vi "AutoRunEngine.vi"(6 "Stop":bool, 7 "Comms in cluster":T3={"Lakeshore port"="COM6", "Lakeshore Error"={"status"=FALSE, "code"=0, "source"=""}, "Cernox Channel"=17, "Sample Channel "=1, "Arduino port \n(for magnetic poles)"="COM3", "Switchboard port"="USB0::0x05E6::0x3706::04089883::INSTR", "Switchboard Error"={"status"=FALSE, "code"=0, "source"=""}, "Hall probe/Aux"=FALSE} {"Cernox Channel" items=["1"=1, "2"=2, "3"=3, "4"=4, "5"=5, "6"=6, "7"=7, "8"=8, "9"=9, "10"=10, "11"=11, "12"=12, "13"=13, "14"=14, "15"=15, "16"=16, "A"=17]; "Sample Channel" items=["1"=1, "2"=2, "3"=3, "4"=4, "5"=5, "6"=6, "7"=7, "8"=8, "9"=9, "10"=10, "11"=11, "12"=12, "13"=13, "14"=14, "15"=15, "16"=16, "A (Control Input)"=17]}, 8 "Save Data":bool, 9 "File path":path) -> (1 "Comms out cluster":T1={"Lakeshore port"="COM6", "Lakeshore Error"={"status"=FALSE, "code"=0, "source"=""}, "Cernox Channel"="", "Sample Channel "="", "Arduino port \n(for magnetic poles)"="COM3", "Switchboard port"="USB0::0x05E6::0x3706::04089883::INSTR", "Switchboard Error 2"={"status"=FALSE, "code"=0, "source"=""}}, 2 "Graph indices out":dbl[](array[numeric]), 3 "Array":dbl[][](array[numeric]))   [LabVIEW 2017, in "Fridge Software v2.1.lvlib"]
uses:
  Fridge Software v2.1.lvlib
  <vilib>/Platform/TimedLoop/XDataNode/timing_clust.ctl
  <vilib>/Platform/TimedLoop/XDataNode/nitl_modes.ctl
  <vilib>/Platform/TimedLoop/XDataNode/wakeup.ctl
  <vilib>/Utility/file.llb/Write Delimited Spreadsheet (DBL).vi
  <vilib>/platform/TimedLoop/XDataNode/XDataNode.xnode
  <instrlib>/Lake Shore 372/Lake Shore 372.lvlib
  <instrlib>/Keithley 3706/Keithley 3700 Series.lvlib
  <vilib>/Platform/TimedLoop/XDataNode/XDNodeRunTimeDep.lvlib
panel:
  out "Input Reading Status Query":string
  out "Elapsed time":dbl=500.0 min=50.0 step=100.0
  out "Magnetic Poles \nLive  Voltage":dbl format="%#_5g"
  in  "Measurement\nperiod":i64=500 min=100 step=100
  out "Power Reading":dbl min=0.0 max=0.01 step=1e-05 format="%^.3g"
  out "Sample Reactance":dbl min=0.0 max=63200000.0 step=1e-05 format="%.3g"
  out "Cernox Resistance":dbl min=0.0 max=63200000.0 step=1e-05 format="%.3g"
  in  "R(T,H) tab":enum32{"R(T)", "R(H)"}(tab)
  in  "Clear R(T) graph":bool
  in  "Autoscale R(T)":bool=TRUE caption="Autoscale"
  out "R(T) Graph":cluster{dbl[], dbl[]}(graph)
  in  "Clear H(T) graph":bool
  in  "Autoscale H(T)":bool=TRUE caption="Autoscale"
  out "R(H) Graph":cluster{dbl[], dbl[]}(graph)
  in  "Clear H(t) graph":bool
  in  "Clear T(t) graph":bool
  in  "Clear R(t) graph":bool
  out "Sample Resistance":dbl min=0.0 max=63200000.0 step=1e-05 format="%^.5g"
  out "Cernox Temperature":dbl min=0.0 max=1000.0 step=1e-05 format="%.4f"
  in  "Autoscale H(t)":bool=TRUE caption="Autoscale"
  in  "Autoscale T(t)":bool=TRUE caption="Autoscale"
  in  "Autoscale R(t)":bool=TRUE caption="Autoscale"
  out "H(t) Graph 4":cluster{dbl[], dbl[]}(graph)
  out "T(t) Graph 3":cluster{dbl[], dbl[]}(graph)
  out "R(t) Graph":cluster{dbl[], dbl[]}(graph)
  in  "Measurement":T2(tab)
  in  "Update":bool
  out "Excitation  Ind":bool=TRUE
  out "Excitation Mode Ind":u16(ring)=1 items=["Voltage", "Current"]
  out "Excitation Range Ind":u16(ring)=19 items=["31.6 mA"=22, "10.0 mA"=21, "3.16 mA"=20, "1.00 mA"=19, "316 uA"=18, "100 uA"=17, "31.6 uA"=16, "10.0 uA"=15, "3.16 uA"=14, "1.00 uA"=13, "632 mV / 316 nA"=12, "200 mV / 100 nA"=11, "63.2 mV / 31.6 nA"=10, "20.0 mV / 10.0 nA"=9, "6.32 mV / 3.16 nA"=8, "2.00 mV / 1.00 nA"=7, "632 uV / 316 pA"=6, "200 uV / 100 pA"=5, "63.2 uV / 31.6 pA"=4, "20.0 uV / 10.0 pA"=3, "6.32 uV / 3.16 pA"=2, "2.00 uV / 1.00 pA"=1]
  out "Autorange Ind":u16(ring) items=["Autorange off", "Autorange Current", "ROX 102B Autorange"]
  out "Resistance Range Ind":u16(ring)=8 items=["63.2 MOhm"=22, "20.0 MOhm"=21, "6.32 MOhm"=20, "2.00 MOhm"=19, "632 kOhm"=18, "200 kOhm"=17, "63.2 kOhm"=16, "20.0 kOhm"=15, "6.32 kOhm"=14, "2.00 kOhm"=13, "632 Ohm"=12, "200 Ohm"=11, "63.2 Ohm"=10, "20.0 Ohm"=9, "6.32 Ohm"=8, "2.00 Ohm"=7, "632 mOhm"=6, "200 mOhm"=5, "63.2 mOhm"=4, "20.0 mOhm"=3, "6.32 mOhm"=2, "2.00 mOhm"=1]
  out "Preferred Units Ind":u16(ring)=2 items=["Kelvin"=1, "Ohms"=2]
  out "Temperature Limit Ind":dbl min=0.0 max=2999.0 step=1.0
  in  "Excitation Mode":u16(ring)=1 items=["Voltage", "Current"]
  in  "Excitation Range":u16(ring)=19 items=["31.6 mA"=22, "10.0 mA"=21, "3.16 mA"=20, "1.00 mA"=19, "316 uA"=18, "100 uA"=17, "31.6 uA"=16, "10.0 uA"=15, "3.16 uA"=14, "1.00 uA"=13, "632 mV / 316 nA"=12, "200 mV / 100 nA"=11, "63.2 mV / 31.6 nA"=10, "20.0 mV / 10.0 nA"=9, "6.32 mV / 3.16 nA"=8, "2.00 mV / 1.00 nA"=7, "632 uV / 316 pA"=6, "200 uV / 100 pA"=5, "63.2 uV / 31.6 pA"=4, "20.0 uV / 10.0 pA"=3, "6.32 uV / 3.16 pA"=2, "2.00 uV / 1.00 pA"=1]
  in  "Autorange (0: Autorange off)":u16(ring) items=["Autorange off", "Autorange Current", "ROX 102B Autorange"]
  in  "Resistance Range":u16(ring)=8 items=["63.2 MOhm"=22, "20.0 MOhm"=21, "6.32 MOhm"=20, "2.00 MOhm"=19, "632 kOhm"=18, "200 kOhm"=17, "63.2 kOhm"=16, "20.0 kOhm"=15, "6.32 kOhm"=14, "2.00 kOhm"=13, "632 Ohm"=12, "200 Ohm"=11, "63.2 Ohm"=10, "20.0 Ohm"=9, "6.32 Ohm"=8, "2.00 Ohm"=7, "632 mOhm"=6, "200 mOhm"=5, "63.2 mOhm"=4, "20.0 mOhm"=3, "6.32 mOhm"=2, "2.00 mOhm"=1]
  in  "Preferred Units (2: Ohms)":u16(ring)=2 items=["Kelvin"=1, "Ohms"=2]
  in  "Temperature Limit (0 Kelvin)":dbl min=0.0 max=2999.0 step=1.0
  in  "Excitation  (T: On)":bool=TRUE caption="On\n\nOff"
  in  "Grab settings":bool
  in  "Heater Setpoint":dbl
  out "Heater Setpoint Ind":string
  in  "Grab Heater settings":bool
  in  "Update Heater Settings":bool
  in  "I+":i32 min=0 max=24 step=1
  in  "I-":i32 min=0 max=24 step=1
  in  "V+":i32 min=0 max=24 step=1
  in  "V-":i32 min=0 max=24 step=1
  in  "Close pins (safe)":bool caption="Close I-V pins -> Lift ground -> Lift common -> Current on"
  in  "Lift pins (safe)":bool caption="Current off -> Common closed -> Ground -> Lift I-V pins"
  in  "Channel Open/Close Array":string
  in  "Open":bool
  in  "Close":bool
  in  "Open All IV":bool
  out "Closed Channels":string
  out "Ground closed":bool
  out "Common rail \nclosed":bool
  out "Common-ground \nlink closed":bool
  in  "Append file":bool
  in  "Aux max voltage (mV)":dbl
  in  "Aux Field Range (Oe)":dbl
  # "Created by Daniel Bromley & Alex Wright, IPF Ltd 2021"
  # "Lakeshore - Measurement"
  # "Channels:"
  # "Keithley - Switchboard"
  # "s"
  # "V"
  # "ms"
  # "W"
  # "jW"
  # "W"
  # "W"
  # "K"
  # "Lakeshore - Measurement"
  # "Channels:"
  # "Keithley - Switchboard"
  # "Hall probe"
  # "Aux"
  # "Excitation Mode"
  # "Excitation Range"
  # "Autorange"
  # "Resistance Range"
  # "Preferred Units"
  # "Temperature Limit"
  # "Excitation"
  # "IV pins"
  # "Array"
  # "Set Filename and Path"
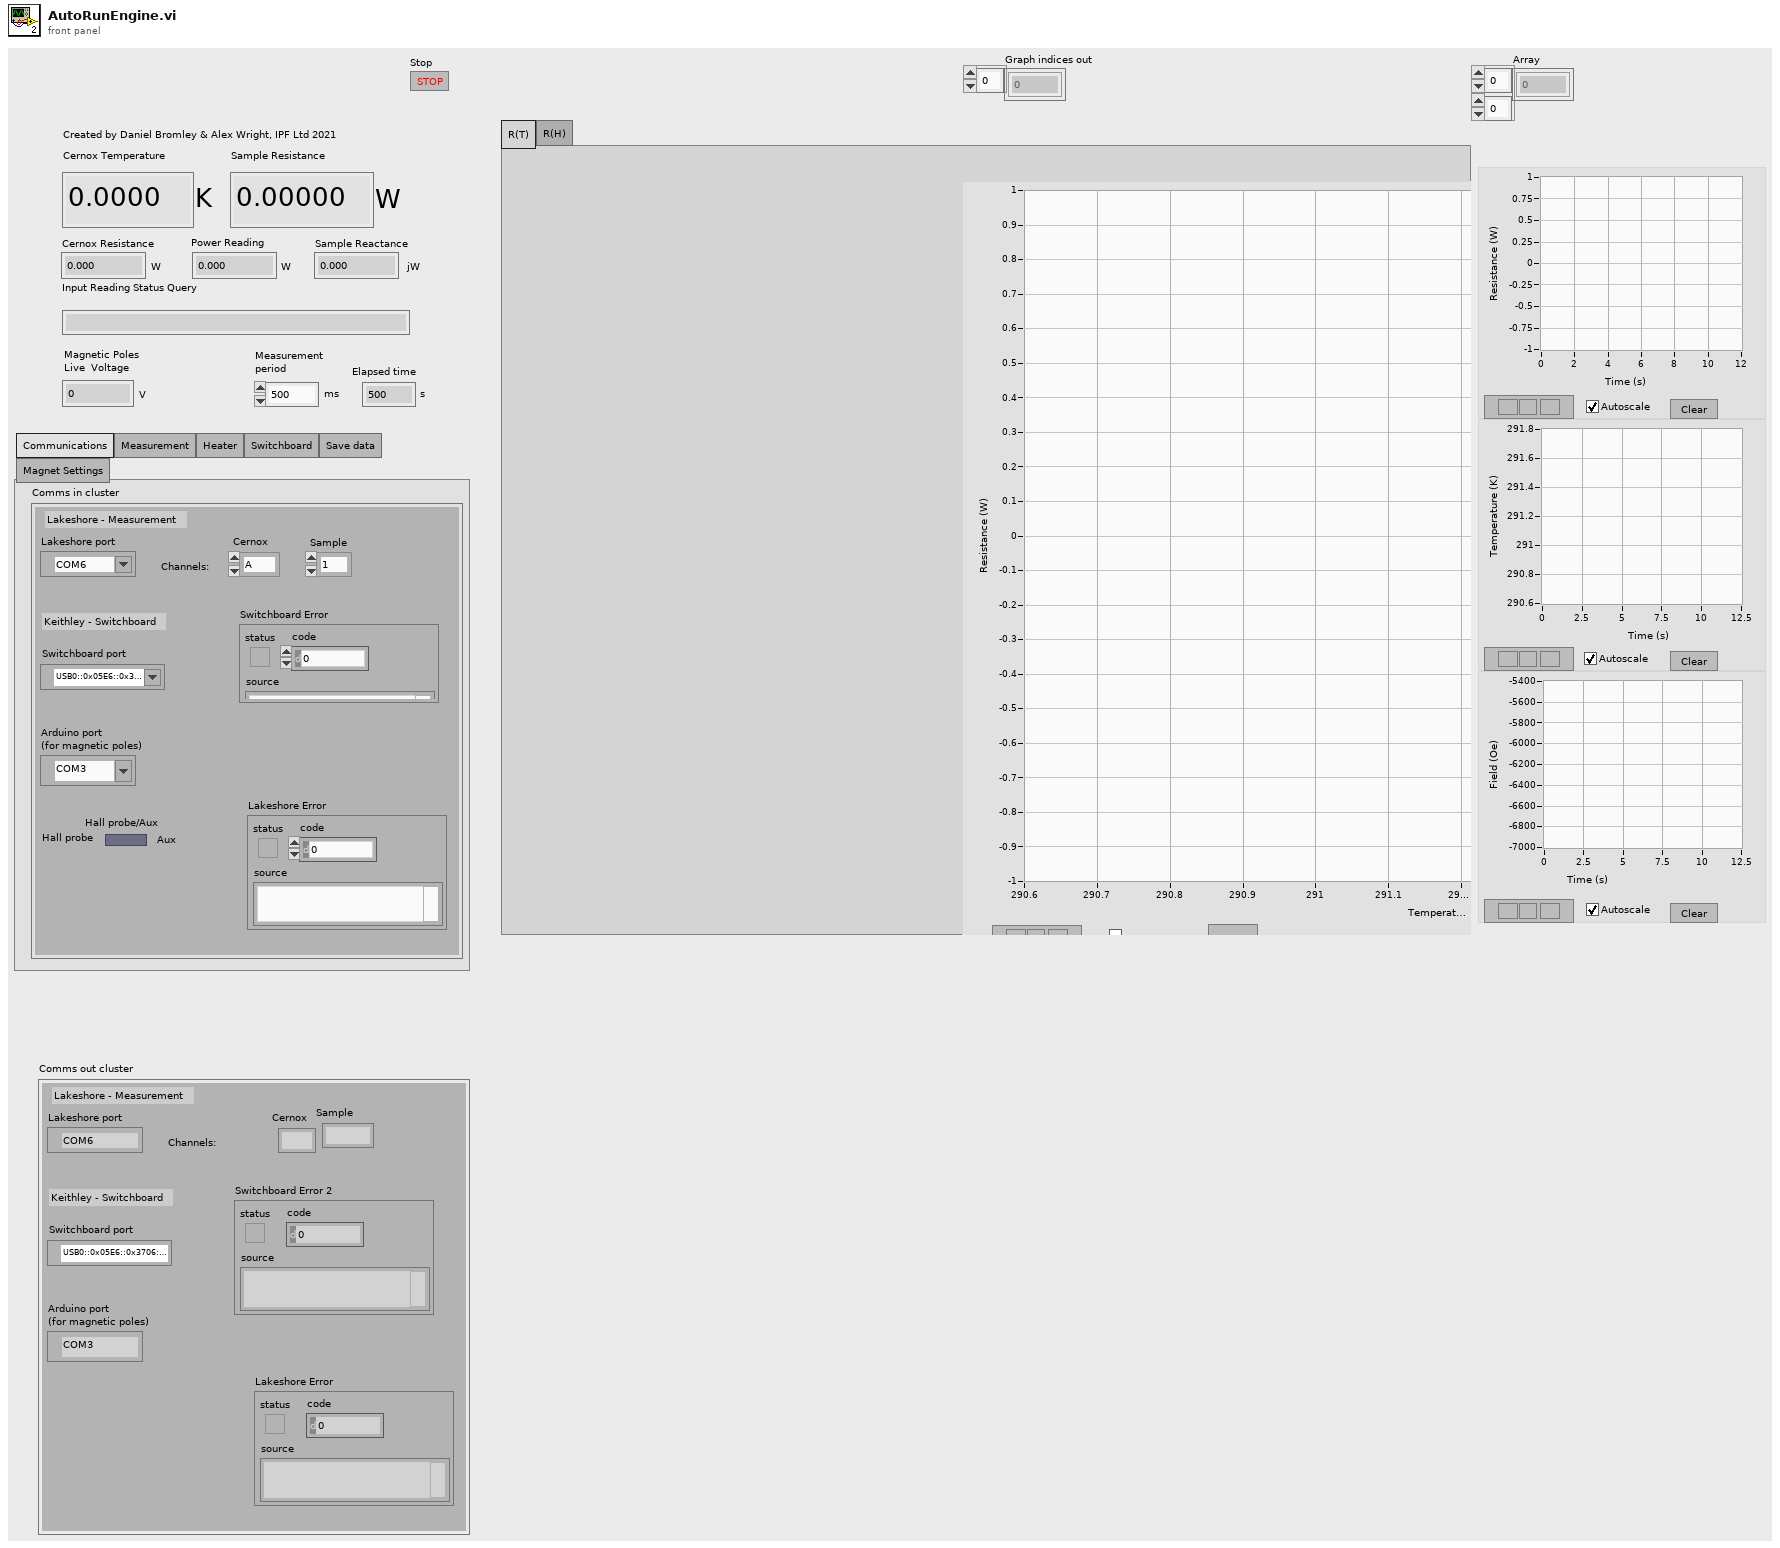
[diagram p1: front panel]
types:
  T1 = cluster{"Lakeshore port":refnum<visa-resource-name>, "Lakeshore Error":errorcluster, "Cernox Channel":string, "Sample Channel ":string, "Arduino port \n(for magnetic poles)":refnum<visa-resource-name>, "Switchboard port":refnum<visa-resource-name>, "Switchboard Error 2":errorcluster}
  T2 = enum32{"Communications", "Measurement", "Heater", "Switchboard", "Save data", "Magnet Settings"}
  T3 = cluster{"Lakeshore port":refnum<visa-resource-name>, "Lakeshore Error":errorcluster, "Cernox Channel":u16, "Sample Channel ":u16, "Arduino port \n(for magnetic poles)":refnum<visa-resource-name>, "Switchboard port":refnum<visa-resource-name>, "Switchboard Error":errorcluster, "Hall probe/Aux":bool}
  T4 = typedef "XDNodeRunTimeDep.lvlib/timing_clust.ctl" = cluster{"Expected End [f-1]":u64, "Actual End [f-1]":u64, "Finished Late? [f-1]":bool, "Expected End [i-1]":u64, "Actual End [i-1]":u64, "Finished Late? [i-1]":bool, "Expected Start [i]":u64, "Actual Start [i]":u64, "Expected Start [f]":u64, "Actual Start [f]":u64, "Source Name":string, "Structure Name":string, "Period":i64, "Deadline":i64, "Offset":i64, "Start":i64, "Priority":i32, "Timeout":i32, "Mode":T5, "Wakeup Reason":T6, "Error":errorcluster, "Source Type":string, "Secondary Source Type":string, "Global End Time":u64, "Global Start Time":u64, "Frame Duration":u64, "Iteration Duration":u64, "Assigned CPU":i32, "I/O Scan Engine Mode":u32}
  T5 = typedef "XDNodeRunTimeDep.lvlib/nitl_modes.ctl" = enum32{"No Change", "Process missed periods, maintain original phase", "Discard missed periods, maintain original phase", "Process missed periods, ignore original phase", "Discard missed periods, ignore original phase"}
  T6 = typedef "XDNodeRunTimeDep.lvlib/wakeup.ctl" = enum32{"Normal", "Aborted", "Asynchronous wakeup", "Timing source error", "Timed loop error", "Timeout"}
  T7 = typedef "eventsource.ctl" = u32
  T8 = typedef "lveventtype.ctl" = enum32{"Null", "Timeout", "Annotation Menu Selection", "Annotation Menu Selection?", "App Instance Close", "App Instance Close?", "Autoscale Range Change", "Bookmark Info Change", "Cell Edit", "Cell Edit?", "Cursor Grab", "Cursor Grab?", "Cursor Menu Selection", "Cursor Menu Selection?", "Cursor Move", "Cursor Release", "Data Change", "Direction Change", "Display State Change", "Drag Ended", "Drag Enter", "Drag Leave", "Drag Over", "Drag Source Update", "Drag Starting", "Drag Starting?", "Drop", "Exec State Change", "Key Down", "Key Down?", "Key Repeat", "Key Repeat?", "Key Up", "Listbox Double Click", "Menu Activation?", "Menu Selection (App)", "Menu Selection? (App)", "Menu Selection (User)", "Mouse Down", "Mouse Down?", "Mouse Enter", "Mouse Leave", "Mouse Move", "Mouse Up", "Mouse Wheel", "NI Security User Change (App)", "Pane Size", "Panel Close", "Panel Close?", "Panel Resize", "Plot Attribute Change", "Scale Range Change", "Shortcut Menu Activation?", "Shortcut Menu Selection (App)", "Shortcut Menu Selection? (App)", "Shortcut Menu Selection (User)", "Tree Double Click", "Tree Drag", "Tree Drag?", "Tree Drop", "Tree Drop?", "Tree Item Close", "Tree Item Close?", "Tree Item Open", "Tree Item Open?", "User Event", "Value Change"}
  T9 = cluster{"VISA Refnum out":refnum<visa-resource-name>, "error out":errorcluster, "Channel Str":string, "Channel Str":string, "VISA Refnum out":refnum<visa-resource-name>, "VISA resource name out":refnum<visa-resource-name>, "error out":errorcluster}
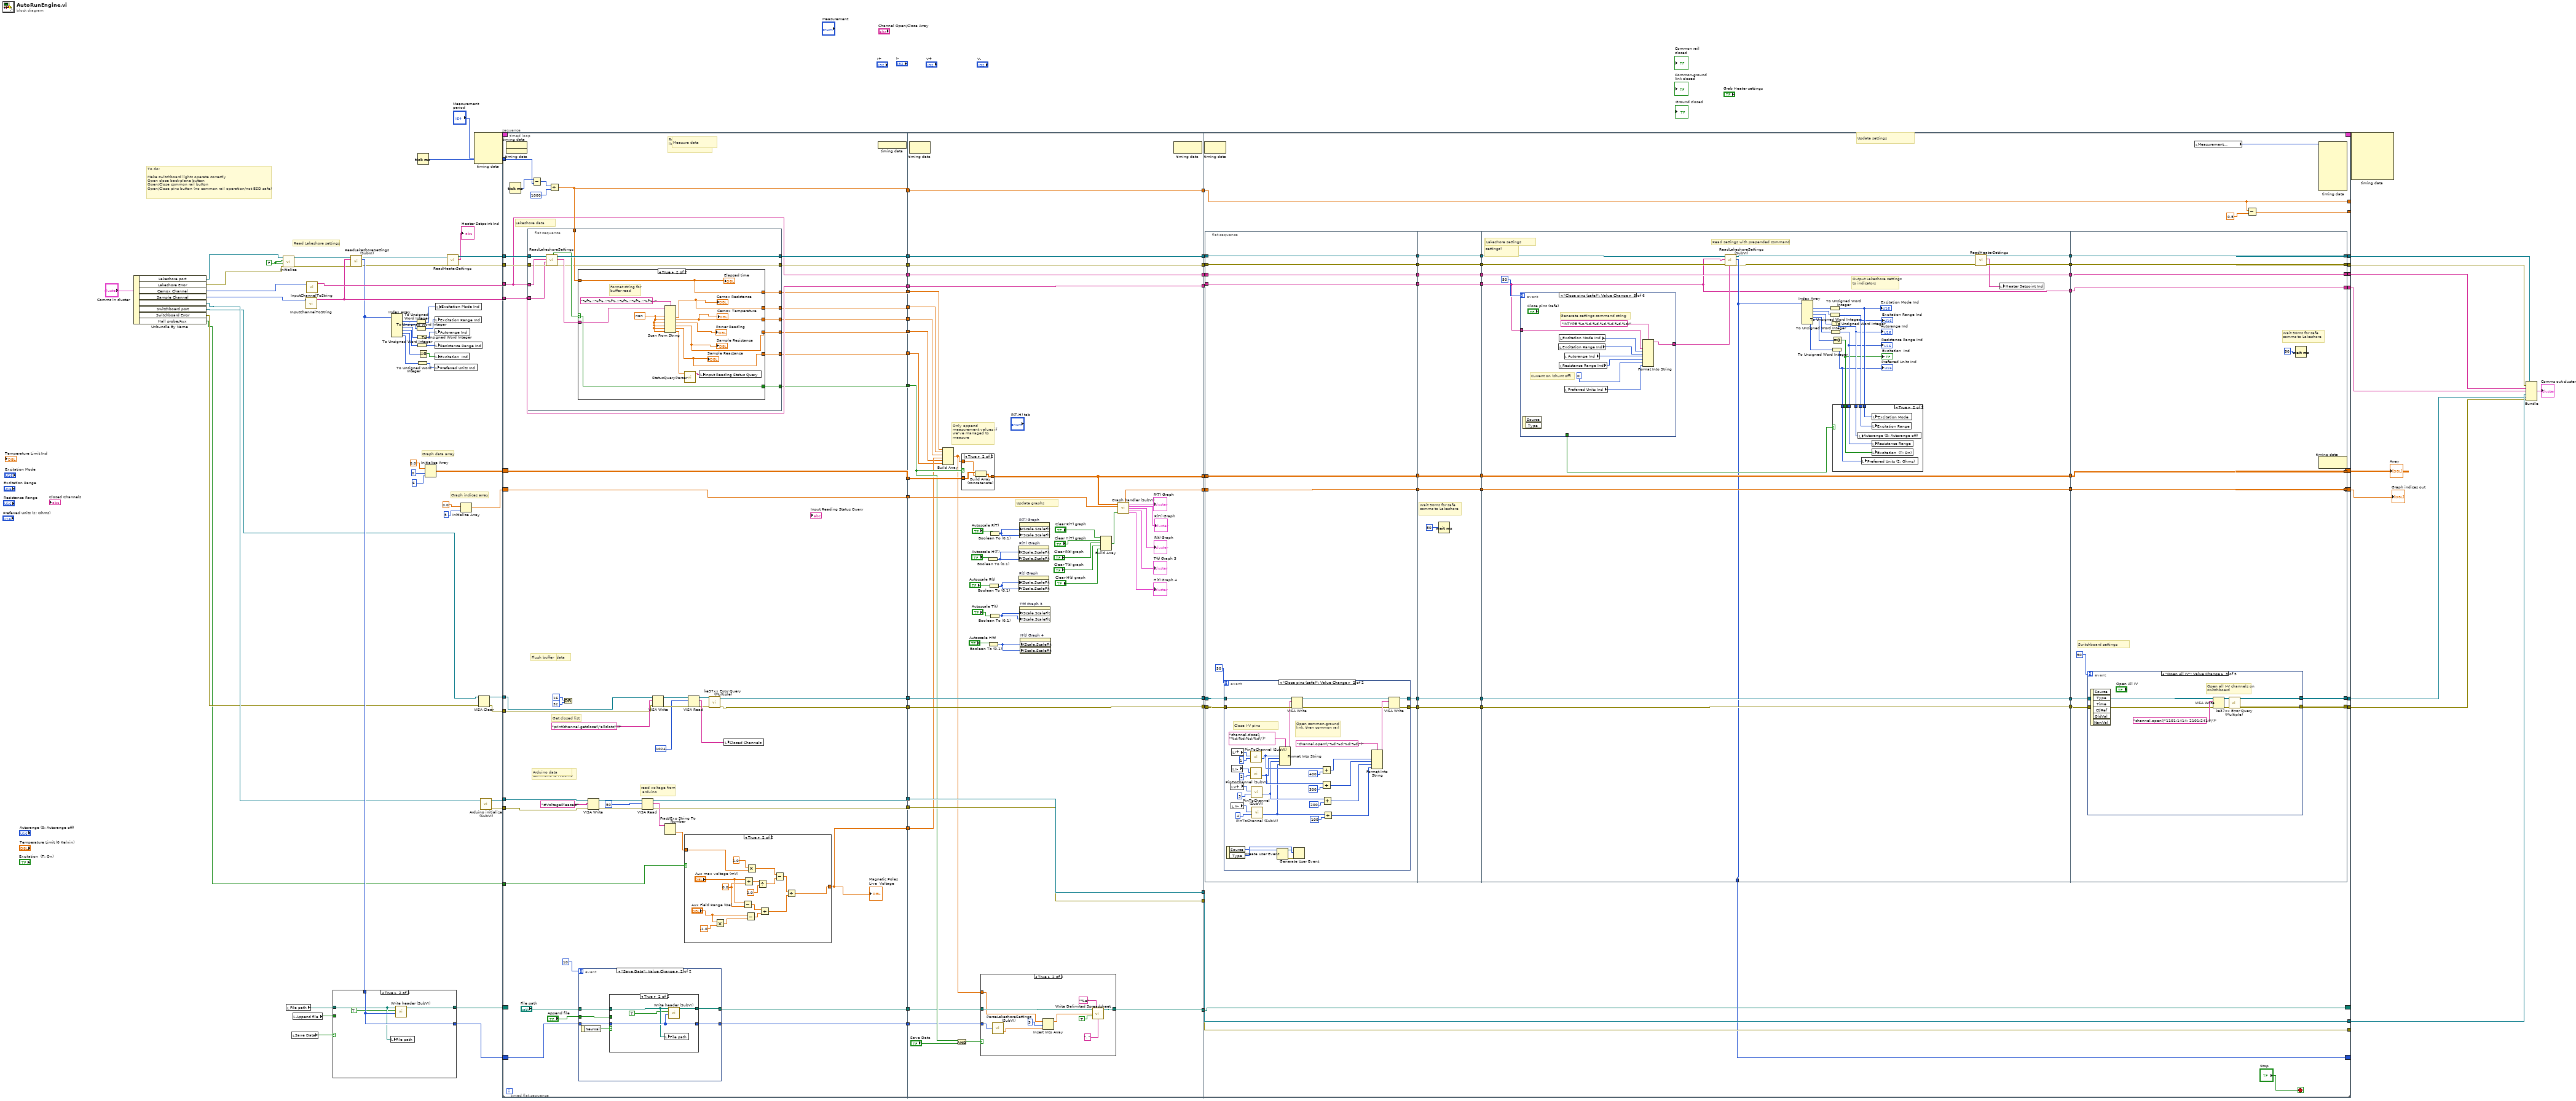
[diagram p0: block diagram]
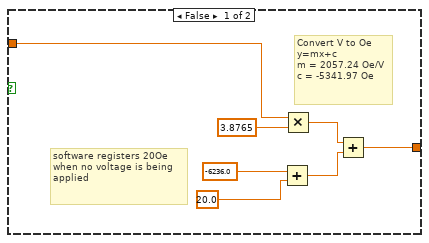
[diagram p3: hidden frame]
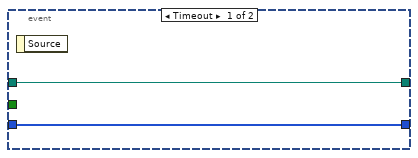
[diagram p4: hidden frame]
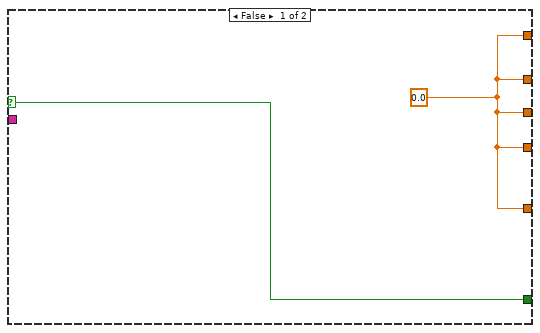
[diagram p6: hidden frame]
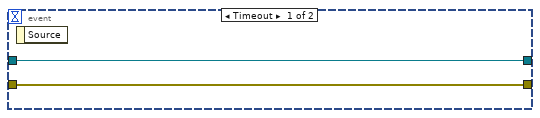
[diagram p9: hidden frame]
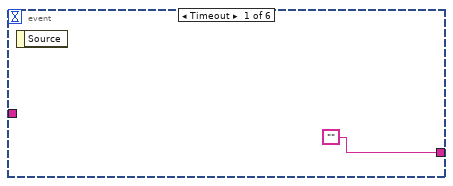
[diagram p10: hidden frame]
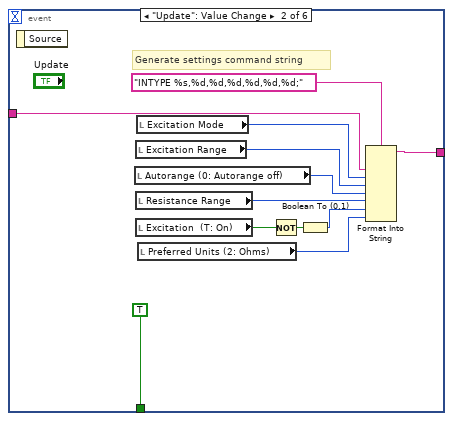
[diagram p11: hidden frame]
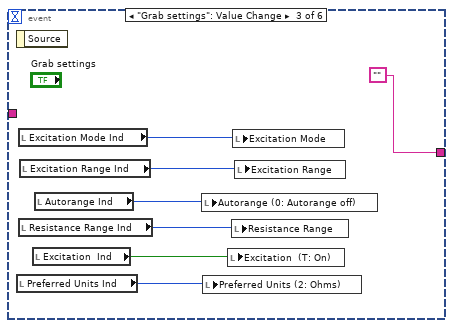
[diagram p12: hidden frame]
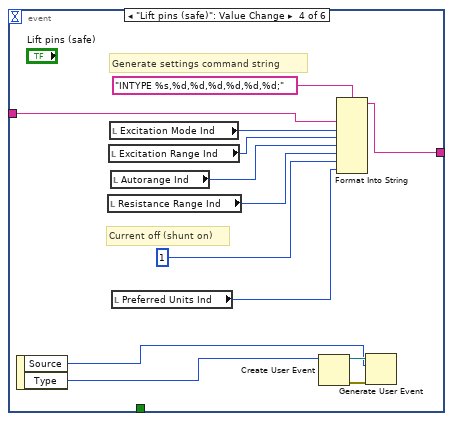
[diagram p13: hidden frame]
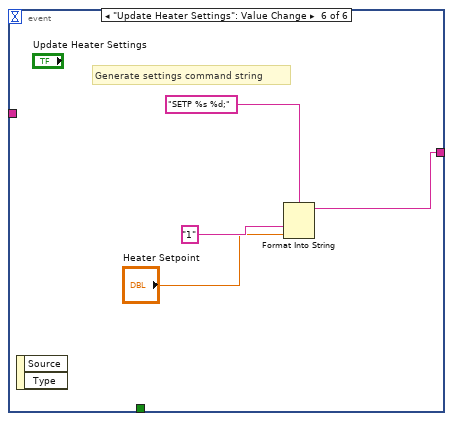
[diagram p14: hidden frame]
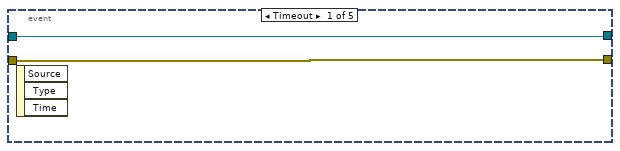
[diagram p16: hidden frame]
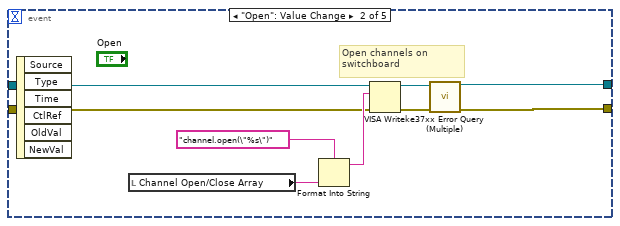
[diagram p17: hidden frame]
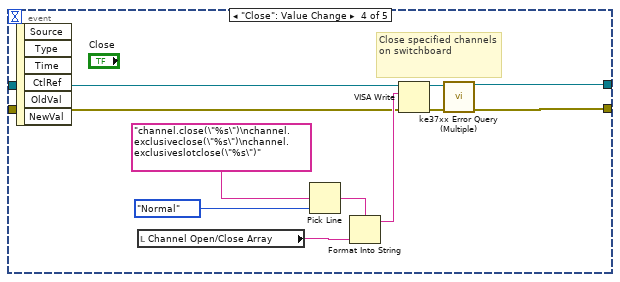
[diagram p18: hidden frame]
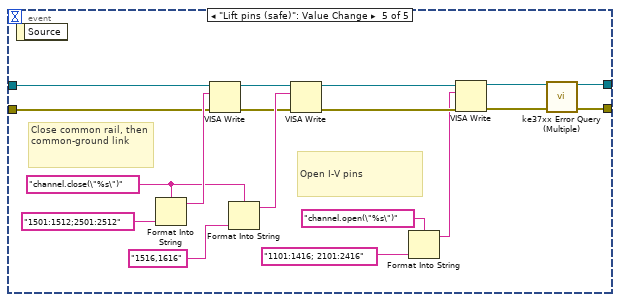
[diagram p19: hidden frame]
diagram:
  w27 = FALSE
  # "To do:\n\nMake switchboard lights operate correctly\nOpen close back-plane button\nOpen/Close common rail button\nOpen/Close pins button (no common rail operation/not ESD safe)"
  # "Read Lakeshore settings"
  # "Graph indices array"
  # "Graph data array"
  n1 = Unbundle By Name("Comms in cluster") -> ("Lakeshore port"=w17:refnum<visa-resource-name>, "Lakeshore Error"=w16:errorcluster, "Cernox Channel"=w15:u16, "Sample Channel"=w14:u16, "Arduino port \n(for magnetic poles)"=w13:refnum<visa-resource-name>, "Switchboard port"=w12:refnum<visa-resource-name>, "Switchboard Error"=w11:errorcluster, "Hall probe/Aux"=w10:bool)
  n2 = call <instrlib>:"Initialize.vi"("error in (no error)"=w16, "Reset (True)"=w27, "ID Query (True)"=w27, "VISA resource name"=w17) -> ("error out"=w26:errorcluster, "VISA resource name out"=w44:refnum<visa-resource-name>)  [unwired: 6 in]
  n3 = local read "File path"() -> (w28:path)
  n4 = local read "Save Data"() -> (w39:bool)
  n5 = local read "Append file"() -> (w38:bool)
  n6 = call <instrlib>:"InputChannelToString.vi"("Channel (1)"=w14) -> ("Channel Str"=w42:string)  [unwired: 10 in]
  n7 = call <instrlib>:"InputChannelToString.vi"("Channel (1)"=w15) -> ("Channel Str"=w43:string)  [unwired: 10 in]
  n8 = call "ReadLakeshoreSettings (SubVI).vi"("error in (no error)"=w26, "Channel Str"=w42, "Lakeshore port"=w44) -> ("error out"=w23:errorcluster, "Settings array out"=w37:i32[], "VISA Refnum out"=w25:refnum<visa-resource-name>)  [unwired: 4 in]
  n9 = case shown="True" w39 {
    tunnel: w38 -> [_ _]
    tunnel: w37 -> [w64 w68]
    tunnel: [w64 w68] -> w36
    tunnel: [w63 w67] -> w29
    tunnel: w28 -> [w63 w66]
    frame False {
    }
    frame True {
      n10 = local write "File path"(w66) -> ()
      n11 = call "Write header (SubVI).vi"("Settings array in"=w68, "Append? Out"=TRUE, "Path in"=w66) -> ("Path out"=w67:path)  [unwired: 8 in]
    }
  }
  n12 = Index Array(array=w37) -> (element #1=w50:i32, element #2=w49:i32, element #3=w48:i32, element #4=w47:i32, element #5=w46:i32, element #6=w45:i32)  [unwired: 6 in]
  n13 = To Unsigned Word Integer(number=w50) -> (unsigned 16bit integer=w35:u16)
  n14 = To Unsigned Word Integer(number=w49) -> (unsigned 16bit integer=w34:u16)
  n15 = To Unsigned Word Integer(number=w47) -> (unsigned 16bit integer=w32:u16)
  n16 = To Unsigned Word Integer(number=w48) -> (unsigned 16bit integer=w33:u16)
  n17 = To Unsigned Word Integer(number=w45) -> (unsigned 16bit integer=w30:u16)
  n18 = Tick Count (ms)() -> (millisecond timer value=w62:u32)
  n19 = Equal To 0?(x=w46) -> (x = 0?=w31:bool)
  n20 = Initialize Array(0.0, 0, 6) -> (w54:dbl[][])
  n21 = local write "Preferred Units Ind"(w30) -> ()
  n22 = local write "Excitation Range Ind"(w34) -> ()
  n23 = local write "Autorange Ind"(w33) -> ()
  n24 = local write "Resistance Range Ind"(w32) -> ()
  n25 = local write "Excitation  Ind"(w31) -> ()
  n26 = local write "Excitation Mode Ind"(w35) -> ()
  n27 = call "ReadHeaterSettings.vi"("error in (no error)"=w23, "VISA Refnum in"=w25) -> ("error out"=w22:errorcluster, "read buffer"=→"Heater Setpoint Ind":string, "VISA Refnum out"=w24:refnum<visa-resource-name>)  [unwired: 7 in]
  n28 = Initialize Array(0.0, 5) -> (w51:dbl[])
  n29 = node-c288("Measurement\nperiod") -> (w61:T4)  [unwired: 3 in]
  n30 = VISA Clear(VISA resource name=w12, error in (no error)=w11) -> (VISA resource name out=w58:refnum<visa-resource-name>, error out=w9:errorcluster)
  n31 = call "Arduino initialize (SubVI).vi"("VISA Refnum in"=w13) -> ("error out"=w40:errorcluster, "VISA Refnum out"=w41:refnum<visa-resource-name>)  [unwired: 9 in]
  n32 = timed-loop {
    timing: w61 -> [_]
    timing-out: [_] -> w60
    tunnel: w43 -> [w96]
    tunnel: w42 -> [w95]
    tunnel: w22 -> [w94]
    tunnel: w24 -> [w93]
    tunnel: w41 -> [w92]
    tunnel: w40 -> [w91]
    tunnel: [w90] -> w8
    tunnel: [w89] -> w7
    tunnel: [w88] -> w4
    tunnel: [w87] -> _
    tunnel: w58 -> [w86]
    tunnel: w62 -> [w85]
    tunnel: [w84] -> w3
    tunnel: [w83] -> w2
    shift-right: [w82] -> w20
    shift-left: w54 -> [w81]
    shift-right: [w80] -> w19
    shift-left: w51 -> [w79]
    tunnel: [w78] -> _
    tunnel: [w77] -> _
    shift-right: [w76] -> _
    shift-left: w36 -> [w75]
    shift-right: [w74] -> _
    shift-left: w29 -> [w73]
    tunnel: w10 -> [w72]
    tunnel: w9 -> [w71]
    tunnel: [w70] -> w6
    tunnel: [w69] -> w5
    stop <- "Stop" stop-if-true
    n33 = timed-sequence {
      timing: _ -> [_]
      timing-out: _ -> [_]
      tunnel: w96 -> [w153]
      tunnel: w95 -> [w156]
      tunnel: w94 -> [w155]
      tunnel: w93 -> [w154]
      tunnel: w92 -> [w148]
      tunnel: w91 -> [w147]
      tunnel: [w152] -> w90
      tunnel: [w151] -> w89
      tunnel: [w150] -> w88
      tunnel: [w149] -> w87
      tunnel: w86 -> [w146]
      tunnel: w85 -> [w145]
      tunnel: [w144] -> w84
      tunnel: [w143] -> w83
      tunnel: [w142] -> w82
      tunnel: w81 -> [w141]
      tunnel: [w115] -> w80
      tunnel: w79 -> [w113]
      tunnel: [w111] -> w78
      tunnel: [w110] -> w77
      tunnel: [w109] -> w76
      tunnel: w75 -> [w108]
      tunnel: [w107] -> w74
      tunnel: w73 -> [w106]
      tunnel: w72 -> [w102]
      tunnel: w71 -> [w101]
      tunnel: [w98] -> w70
      tunnel: [w97] -> w69
      n34 = timed-flat-sequence {
        tunnel: w156 -> [w204]
        tunnel: [w206] -> w140
        tunnel: [w205] -> w138
        tunnel: [w204] -> w136
        tunnel: w155 -> [w203]
        tunnel: w154 -> [w202]
        tunnel: w153 -> [w157]
        tunnel: [w198] -> w134
        tunnel: [w197] -> w132
        tunnel: w148 -> [w183]
        tunnel: w147 -> [w182]
        tunnel: w146 -> [w184]
        tunnel: [w169] -> w130
        tunnel: [w168] -> w128
        tunnel: w145 -> [w180]
        tunnel: [w171] -> w126
        tunnel: w141 -> [w179]
        tunnel: [w179] -> w124
        tunnel: [w178] -> w123
        tunnel: [w177] -> w122
        tunnel: [w176] -> w121
        tunnel: [w175] -> w120
        tunnel: [w174] -> w119
        tunnel: [w160] -> w118
        tunnel: [w173] -> w116
        tunnel: [w172] -> w114
        tunnel: w113 -> [w172]
        tunnel: w108 -> [w167]
        tunnel: w106 -> [_]
        tunnel: [w163] -> w105
        tunnel: [w162] -> w103
        tunnel: w102 -> [w159]
        tunnel: w101 -> [w158]
        tunnel: [w157] -> w100
        tunnel: w140 -> [w321]
        tunnel: [w321] -> w139
        tunnel: w138 -> [w320]
        tunnel: [w320] -> w137
        tunnel: w136 -> [w319]
        tunnel: [w319] -> w135
        tunnel: w134 -> [w318]
        tunnel: [w318] -> w133
        tunnel: w132 -> [w317]
        tunnel: [w317] -> w131
        tunnel: w130 -> [w316]
        tunnel: [w316] -> w129
        tunnel: w128 -> [w315]
        tunnel: [w315] -> w127
        tunnel: w126 -> [w314]
        tunnel: [w314] -> w125
        tunnel: w124 -> [w313]
        tunnel: w123 -> [w312]
        tunnel: w122 -> [w311]
        tunnel: w121 -> [w310]
        tunnel: w120 -> [w277]
        tunnel: w119 -> [w276]
        tunnel: w118 -> [w278]
        tunnel: [w294] -> w117
        tunnel: w116 -> [w284]
        tunnel: w114 -> [w293]
        tunnel: [w291] -> w112
        tunnel: w105 -> [w281]
        tunnel: [w280] -> w104
        tunnel: w103 -> [w279]
        tunnel: w100 -> [w275]
        tunnel: [w275] -> w99
        tunnel: w139 -> [w387]
        tunnel: w137 -> [w386]
        tunnel: w135 -> [w385]
        tunnel: [w384] -> w152
        tunnel: [w383] -> w151
        tunnel: w133 -> [w382]
        tunnel: w131 -> [w381]
        tunnel: [w382] -> w150
        tunnel: [w381] -> w149
        tunnel: w129 -> [w376]
        tunnel: w127 -> [w375]
        tunnel: w125 -> [w349]
        tunnel: [w378] -> w144
        tunnel: [w377] -> w143
        tunnel: [w356] -> w142
        tunnel: w117 -> [w358]
        tunnel: [w351] -> w115
        tunnel: w112 -> [w354]
        tunnel: [w349] -> w111
        tunnel: [w348] -> w110
        tunnel: [w347] -> w109
        tunnel: [w346] -> w107
        tunnel: w104 -> [w346]
        tunnel: w99 -> [w345]
        tunnel: [w340] -> w98
        tunnel: [w339] -> w97
        frame #0 {
          # "Request and read closed list from switchboard"
          # "Get closed list"
          # "Flush buffer"
          # "Switchboard data"
          # "Arduino data"
          # "Lakeshore data"
          # "read voltage from\n arduino"
          # "Write voltage read command to Arduino"
          # "Measure data"
          n35 = node-c288() -> ()  [unwired: 1 in]
          n36 = Tick Count (ms)() -> (millisecond timer value=w181:u32)
          n37 = flat-sequence {
            tunnel: w204 -> [w252]
            tunnel: w203 -> [w256]
            tunnel: w202 -> [w255]
            tunnel: w157 -> [w257]
            tunnel: [w258] -> w206
            tunnel: [w244] -> w205
            tunnel: w171 -> [w251]
            tunnel: [w250] -> w178
            tunnel: [w249] -> w177
            tunnel: [w248] -> w176
            tunnel: [w247] -> w175
            tunnel: [w246] -> w174
            tunnel: [w245] -> w173
            frame #0 {
              n38 = call "ReadLakeshoreSettings.vi"("error in (no error)"=w256, "Sample Channel Str"=w252, "Cernox channel string"=w257, "VISA Refnum in"=w255) -> ("error out"=w244:errorcluster, "Read output"=w254:string, "VISA Refnum out"=w258:refnum<visa-resource-name>, "Boolean"=w253:bool)  [unwired: 4 in]
              n39 = case shown="True" w253 {
                selector: w253 -> [w259 w269]
                tunnel: w254 -> [_ w271]
                tunnel: w251 -> [_ w266]
                tunnel: [w260 w266] -> w250
                tunnel: [w260 w264] -> w249
                tunnel: [w260 w263] -> w248
                tunnel: [w260 w261] -> w247
                tunnel: [w260 w265] -> w246
                tunnel: [w259 w269] -> w245
                frame False {
                  w260 = 0.0
                }
                frame True {
                  w270 = nan
                  # "Format string for buffer read"
                  n40 = Scan From String(format string="%f%.;;%f%.;;%f%.;;%f%.;;%f%.;;%f%.;", input string=w271, default 1=w270, default 2=w270, default 3=w270, default 4=w270, default 5=w270, default 6=w270) -> (output 1=w264:dbl, output 2=w263:dbl, output 3=→"Power Reading":dbl, output 4=w261:dbl, output 5=w265:dbl, output 6=w268:dbl)  [unwired: 2 in, 3 out]
                  "Sample Reactance" <- w265
                  "Cernox Resistance" <- w264
                  "Cernox Temperature" <- w263
                  "Sample Resistance" <- w261
                  n41 = call "StatusQueryParser.vi"("Numeric"=w268) -> ("String"=w267:string)  [unwired: 10 in]
                  n42 = local write "Input Reading Status Query"(w267) -> ()
                  "Elapsed time" <- w266
                }
              }
            }
          }
          n43 = Subtract(x=w181, y=w180) -> (x-y=w187:u32)
          n44 = Divide(x=w187, y=1000) -> (x/y=w171:dbl)
          n45 = Or(x=16, y=32) -> ()  [unwired: 1 out]
          n46 = event shown="[1] \"Save Data\": Value Change" {
            selector: _ -> [_ _]
            dyn-events: _ -> [_ _]
            timeout: 10 -> [_ _]
            tunnel: w167 -> [w230 w236]
            tunnel: "Append file" -> [_ w235]
            tunnel: "File path" -> [w231 w234]
            tunnel: [w231 w233] -> w163
            tunnel: [w230 w232] -> w162
            event Timeout {
              n47 = event-data() -> ()  [unwired: 1 in, 1 out]
            }
            event "Save Data": Value Change {
              n48 = event-data() -> ("NewVal"=w237:bool)  [unwired: 1 in]
              n49 = case shown="True" w237 {
                tunnel: w236 -> [w238 w242]
                tunnel: w235 -> [_ _]
                tunnel: w234 -> [w239 w241]
                tunnel: [w239 w243] -> w233
                tunnel: [w238 w242] -> w232
                frame False {
                }
                frame True {
                  n50 = local write "File path"(w241) -> ()
                  n51 = call "Write header (SubVI).vi"("Settings array in"=w242, "Append? Out"=TRUE, "Path in"=w241) -> ("Path out"=w243:path)  [unwired: 8 in]
                }
              }
            }
          }
          n52 = VISA Write(VISA resource name=w183, write buffer="#VoltagePlease#" ("Send to Arduino"), error in (no error)=w182) -> (VISA resource name out=w199:refnum<visa-resource-name>, error out=w196:errorcluster)  [unwired: 1 out]
          n53 = VISA Read(VISA resource name=w199, byte count=u32 50 ("milliseconds to wait"), error in (no error)=w196) -> (VISA resource name out=w198:refnum<visa-resource-name>, read buffer=w201:string, error out=w197:errorcluster)  [unwired: 1 out]
          n54 = VISA Write(VISA resource name=w184, write buffer="print(channel.getclose(\"allslots\"))", error in (no error)=w158) -> (VISA resource name out=w193:refnum<visa-resource-name>, error out=w192:errorcluster)  [unwired: 1 out]
          n55 = Fract/Exp String To Number(string=w201) -> (number=w161:dbl)  [unwired: 3 in, 1 out]
          n56 = case shown="True" w159 {
            tunnel: w161 -> [w208 w221]
            tunnel: [w207 w218] -> w160
            frame False {
              # "software registers 20Oe when no voltage is being applied"
              # "Convert V to Oe\ny=mx+c\nm = 2057.24 Oe/V\nc = -5341.97 Oe"
              n57 = Add(x=-6236.0, y=20.0) -> (x+y=w212:dbl)
              n58 = Multiply(x=w208, y=3.8765) -> (x*y=w213:dbl)
              n59 = Add(x=w213, y=w212) -> (x+y=w207:dbl)
            }
            frame True {
              w226 = 0.0
              n60 = Multiply(x="Aux Field Range (Oe)", y=-1.0) -> (x*y=w216:dbl)
              n61 = Subtract(x="Aux max voltage (mV)", y=w226) -> (x-y=w225:dbl)
              n62 = Add(x="Aux max voltage (mV)", y=w226) -> (x+y=w229:dbl)
              n63 = Subtract(x="Aux Field Range (Oe)", y=w216) -> (x-y=w224:dbl)
              n64 = Multiply(x=1.0, y=w221) -> (x*y=w219:dbl)
              n65 = Divide(x=w229, y=2.0) -> (x/y=w227:dbl)
              n66 = Divide(x=w225, y=w224) -> (x/y=w222:dbl)
              n67 = Subtract(x=w219, y=w227) -> (x-y=w223:dbl)
              n68 = Divide(x=w223, y=w222) -> (x/y=w218:dbl)
            }
          }
          "Magnetic Poles \nLive  Voltage" <- w160
          n69 = VISA Read(VISA resource name=w193, byte count=u32 1024 ("Bytes To Read (1024)"), error in (no error)=w192) -> (VISA resource name out=w194:refnum<visa-resource-name>, read buffer=w185:string, error out=w170:errorcluster)  [unwired: 1 out]
          n70 = call <instrlib>:"ke37xx Error Query (Multiple).vi"("VISA resource name"=w194, "error in (no error)"=w170) -> ("VISA resource name out"=w169:refnum<visa-resource-name>, "error out"=w168:errorcluster)  [unwired: 10 in, 2 out]
          n71 = local write "Closed Channels"(w185) -> ()
          n72 = node-c288() -> ()  [unwired: 1 out]
        }
        frame #1 {
          # "Update graphs"
          # "Only append measurement values if we've managed to measure"
          n73 = node-c288() -> ()  [unwired: 1 in, 1 out]
          n74 = Build Array(w312, w311, w310, w278, w277, w276) -> (w282:dbl[])
          n75 = And(x=w284, y="Save Data") -> (x .and. y?=w283:bool)
          n76 = case shown="True" w284 {
            tunnel: w313 -> [w333 w335]
            tunnel: w282 -> [_ w334]
            tunnel: [w333 w336] -> w294
            frame False {
            }
            frame True {
              n77 = Build Array (concatenate)(w335, w334) -> (w336:dbl[][])
            }
          }
          n78 = case shown="True" w283 {
            tunnel: w282 -> [_ w326]
            tunnel: w281 -> [w322 w332]
            tunnel: [w322 w331] -> w280
            tunnel: w279 -> [_ w324]
            frame False {
            }
            frame True {
              n79 = call "ParseLakeshoreSettings (SubVI).vi"("Settings array in"=w324) -> ("Current excitation (A)"=w323:dbl)  [unwired: 1 out]
              n80 = Insert Into Array(array=w326, index=3, new element=w323) -> (w325:dbl[])
              n81 = call-poly <vilib>:"Write Delimited Spreadsheet.vi"("file path (dialog if empty)"=w332, "format (%.3f)"="%e", "1D data"=w325, "append to file? (new file:F)"=TRUE, "delimiter (\\t)"=", ") -> ("new file path (Not A Path if cancelled)"=w331:path)  [unwired: 9 in, 1 out]
            }
          }
          n82 = Boolean To (0,1)(Boolean="Autoscale H(T)") -> (0, 1=w295:i16)
          n83 = Boolean To (0,1)(Boolean="Autoscale H(t)") -> (0, 1=w302:i16)
          n84 = Boolean To (0,1)(Boolean="Autoscale R(t)") -> (0, 1=w306:i16)
          n85 = Boolean To (0,1)(Boolean="Autoscale R(T)") -> (0, 1=w308:i16)
          n86 = Boolean To (0,1)(Boolean="Autoscale T(t)") -> (0, 1=w304:i16)
          n87 = property on="R(H) Graph" class="XYGraph (strict)"("XScale.ScaleFit"=w295, "YScale.ScaleFit"=w295) -> ()  [unwired: 2 in, 2 out]
          n88 = property on="R(t) Graph" class="XYGraph (strict)"("XScale.ScaleFit"=w306, "YScale.ScaleFit"=w306) -> ()  [unwired: 2 in, 2 out]
          n89 = property on="R(T) Graph" class="XYGraph (strict)"("XScale.ScaleFit"=w308, "YScale.ScaleFit"=w308) -> ()  [unwired: 2 in, 2 out]
          n90 = property on="T(t) Graph 3" class="XYGraph (strict)"("XScale.ScaleFit"=w304, "YScale.ScaleFit"=w304) -> ()  [unwired: 2 in, 2 out]
          n91 = property on="H(t) Graph 4" class="XYGraph (strict)"("XScale.ScaleFit"=w302, "YScale.ScaleFit"=w302) -> ()  [unwired: 2 in, 2 out]
          n92 = Build Array("Clear R(T) graph", "Clear H(T) graph", "Clear R(t) graph", "Clear T(t) graph", "Clear H(t) graph") -> (w292:bool[])
          n93 = call "Graph handler (SubVI).vi"("Data in"=w294, "Graph indices in"=w293, "Clear graph Array"=w292) -> ("Graph indices out"=w291:dbl[], "R(T) Graph"=→"R(T) Graph":cluster{dbl[], dbl[]}, "R(H) Graph"=→"R(H) Graph":cluster{dbl[], dbl[]}, "R(t) Graph"=→"R(t) Graph":cluster{dbl[], dbl[]}, "T(t) Graph 3"=→"T(t) Graph 3":cluster{dbl[], dbl[]}, "H(t) Graph 4"=→"H(t) Graph 4":cluster{dbl[], dbl[]})  [unwired: 7 in]
          n94 = node-c288() -> ()  [unwired: 1 in, 1 out]
        }
        frame #2 {
          # "Update settings"
          n95 = node-c288() -> ()  [unwired: 1 in, 1 out]
          n96 = flat-sequence {
            tunnel: w375 -> [w394]
            tunnel: w376 -> [w395]
            tunnel: w385 -> [w396]
            tunnel: w386 -> [w397]
            tunnel: w387 -> [w398]
            tunnel: [w398] -> w370
            tunnel: [w397] -> w368
            tunnel: [w396] -> w366
            tunnel: [w393] -> w364
            tunnel: [w392] -> w362
            tunnel: [w390] -> w359
            tunnel: w358 -> [w390]
            tunnel: [w389] -> w355
            tunnel: w354 -> [w389]
            tunnel: w345 -> [w388]
            tunnel: [w388] -> w343
            tunnel: w370 -> [w443]
            tunnel: [w443] -> w369
            tunnel: w368 -> [w442]
            tunnel: [w442] -> w367
            tunnel: w366 -> [w441]
            tunnel: [w441] -> w365
            tunnel: w364 -> [w440]
            tunnel: [w440] -> w363
            tunnel: w362 -> [w439]
            tunnel: [w439] -> w361
            tunnel: [w437] -> w360
            tunnel: w359 -> [w437]
            tunnel: w355 -> [w436]
            tunnel: [w436] -> w352
            tunnel: [w435] -> w344
            tunnel: w343 -> [w435]
            tunnel: [w447] -> w374
            tunnel: [w448] -> w373
            tunnel: [w469] -> w372
            tunnel: [w468] -> w371
            tunnel: w369 -> [w472]
            tunnel: w367 -> [w458]
            tunnel: w365 -> [w444]
            tunnel: w363 -> [w469]
            tunnel: w361 -> [w468]
            tunnel: w360 -> [w467]
            tunnel: [w467] -> w357
            tunnel: [w466] -> w353
            tunnel: w352 -> [w466]
            tunnel: [w457] -> w347
            tunnel: w344 -> [w445]
            tunnel: [w445] -> w342
            tunnel: [w444] -> w341
            tunnel: [w535] -> w384
            tunnel: w374 -> [w535]
            tunnel: [w527] -> w383
            tunnel: w373 -> [w527]
            tunnel: [w533] -> w378
            tunnel: [w532] -> w377
            tunnel: w372 -> [w531]
            tunnel: w371 -> [w530]
            tunnel: w357 -> [w529]
            tunnel: [w529] -> w356
            tunnel: w353 -> [w528]
            tunnel: [w528] -> w351
            tunnel: w342 -> [w526]
            tunnel: w341 -> [w525]
            tunnel: [w526] -> w340
            tunnel: [w525] -> w339
            frame #0 {
              n97 = event shown="[1] \"Close pins (safe)\": Value Change" {
                selector: _ -> [_ _]
                dyn-events: _ -> [_ _]
                timeout: 50 -> [_ _]
                tunnel: w395 -> [w400 w434]
                tunnel: w394 -> [w399 w433]
                tunnel: [w400 w429] -> w393
                tunnel: [w399 w428] -> w392
                event Timeout {
                  n98 = event-data() -> ()  [unwired: 1 in, 1 out]
                }
                event "Close pins (safe)": Value Change {
                  # "Close I-V pins"
                  # "Open common-ground link, then common rail"
                  n99 = event-data() -> ("Source"=w425:T7, "Type"=w426:T8)  [unwired: 1 in]
                  n100 = local read "V+"() -> (w406:i32)
                  n101 = local read "V-"() -> (w403:i32)
                  n102 = local read "I+"() -> (w411:i32)
                  n103 = local read "I-"() -> (w409:i32)
                  n104 = call "PinToChannel (SubVI).vi"("Pin"=w411, "Slot"=1) -> ("Channel"=w410:i32)  [unwired: 8 in]
                  n105 = call "PinToChannel (SubVI).vi"("Pin"=w409, "Slot"=2) -> ("Channel"=w407:i32)  [unwired: 8 in]
                  n106 = call "PinToChannel (SubVI).vi"("Pin"=w406, "Slot"=3) -> ("Channel"=w404:i32)  [unwired: 8 in]
                  n107 = call "PinToChannel (SubVI).vi"("Pin"=w403, "Slot"=4) -> ("Channel"=w401:i32)  [unwired: 8 in]
                  n108 = Create User Event(user event datatype=w426) -> (user event=w424:refnum<user-event>, error out=w427:errorcluster)  [unwired: 1 in]
                  n109 = Format Into String(format string="channel.close(\"%d;%d;%d;%d\")", w410, w407, w404, w401) -> (resulting string=w431:string)  [unwired: 2 in, 1 out]
                  n110 = VISA Write(VISA resource name=w434, write buffer=w431, error in (no error)=w433) -> (VISA resource name out=w422:refnum<visa-resource-name>, error out=w421:errorcluster)  [unwired: 1 out]
                  n111 = Generate User Event(user event=w424, event data cluster=w425, error in=w427) -> ()  [unwired: 1 in, 2 out]
                  n112 = Add(x=w410, y=400) -> (x+y=w416:i32)
                  n113 = Add(x=w407, y=300) -> (x+y=w415:i32)
                  n114 = Add(x=w404, y=200) -> (x+y=w414:i32)
                  n115 = Add(x=w401, y=100) -> (x+y=w413:i32)
                  n116 = Format Into String(format string="channel.open(\"%d;%d;%d;%d\")", w416, w415, w414, w413) -> (resulting string=w423:string)  [unwired: 2 in, 1 out]
                  n117 = VISA Write(VISA resource name=w422, write buffer=w423, error in (no error)=w421) -> (VISA resource name out=w429:refnum<visa-resource-name>, error out=w428:errorcluster)  [unwired: 1 out]
                }
              }
            }
            frame #1 {
              # "Wait 50ms for safe comms to Lakeshore"
              n118 = Wait (ms)(milliseconds to wait=50) -> ()  [unwired: 1 out]
            }
            frame #2 {
              # "Read settings with prepended command"
              # "Lakeshore settings"
              # "Updating measurement settings?"
              # "Output Lakeshore settings to indicators"
              n119 = event shown="[4] \"Close pins (safe)\": Value Change" {
                selector: _ -> [_ _ _ _ _ _]
                dyn-events: _ -> [_ _ _ _ _ _]
                timeout: 50 -> [_ _ _ _ _ _]
                tunnel: w444 -> [_ w477 _ w497 w512 _]
                tunnel: ["" w475 "" w498 w511 w515] -> w459
                tunnel: [_ TRUE _ _ _ _] -> w470
                event Timeout {
                  n120 = event-data() -> ()  [unwired: 1 in, 1 out]
                }
                event "Update": Value Change {
                  # "Generate settings command string"
                  n121 = event-data() -> ()  [unwired: 1 in, 1 out]
                  n122 = local read "Autorange (0: Autorange off)"() -> (w482:u16)
                  n123 = local read "Excitation Range"() -> (w481:u16)
                  n124 = local read "Resistance Range"() -> (w483:u16)
                  n125 = local read "Excitation  (T: On)"() -> (w478:bool)
                  n126 = local read "Excitation Mode"() -> (w480:u16)
                  n127 = local read "Preferred Units (2: Ohms)"() -> (w485:u16)
                  n128 = Not(x=w478) -> (.not. x?=w479:bool)
                  n129 = Boolean To (0,1)(Boolean=w479) -> (0, 1=w484:i16)
                  n130 = Format Into String(format string="INTYPE %s,%d,%d,%d,%d,%d,%d;", w477, w480, w481, w482, w483, w484, w485) -> (resulting string=w475:string)  [unwired: 2 in, 1 out]
                }
                event "Grab settings": Value Change {
                  n131 = event-data() -> ()  [unwired: 1 in, 1 out]
                  n132 = local read "Preferred Units Ind"() -> (w487:u16)
                  n133 = local read "Excitation Mode Ind"() -> (w492:u16)
                  n134 = local read "Resistance Range Ind"() -> (w489:u16)
                  n135 = local read "Excitation Range Ind"() -> (w491:u16)
                  n136 = local read "Excitation  Ind"() -> (w488:bool)
                  n137 = local read "Autorange Ind"() -> (w490:u16)
                  n138 = local write "Autorange (0: Autorange off)"(w490) -> ()
                  n139 = local write "Preferred Units (2: Ohms)"(w487) -> ()
                  n140 = local write "Excitation  (T: On)"(w488) -> ()
                  n141 = local write "Resistance Range"(w489) -> ()
                  n142 = local write "Excitation Mode"(w492) -> ()
                  n143 = local write "Excitation Range"(w491) -> ()
                }
                event "Lift pins (safe)": Value Change {
                  # "Current off (shunt on)"
                  # "Generate settings command string"
                  n144 = event-data() -> ("Source"=w494:T7, "Type"=w493:T8)  [unwired: 1 in]
                  n145 = local read "Resistance Range Ind"() -> (w501:u16)
                  n146 = local read "Excitation Range Ind"() -> (w503:u16)
                  n147 = local read "Excitation Mode Ind"() -> (w504:u16)
                  n148 = local read "Autorange Ind"() -> (w502:u16)
                  n149 = local read "Preferred Units Ind"() -> (w500:u16)
                  n150 = Create User Event(user event datatype=w493) -> (user event=w495:refnum<user-event>, error out=w496:errorcluster)  [unwired: 1 in]
                  n151 = Format Into String(format string="INTYPE %s,%d,%d,%d,%d,%d,%d;", w497, w504, w503, w502, w501, 1, w500) -> (resulting string=w498:string)  [unwired: 2 in, 1 out]
                  n152 = Generate User Event(user event=w495, event data cluster=w494, error in=w496) -> ()  [unwired: 1 in, 2 out]
                }
                event "Close pins (safe)": Value Change {
                  # "Current on (shunt off)"
                  # "Generate settings command string"
                  n153 = event-data() -> ()  [unwired: 1 in, 2 out]
                  n154 = local read "Excitation Range Ind"() -> (w510:u16)
                  n155 = local read "Excitation Mode Ind"() -> (w513:u16)
                  n156 = local read "Resistance Range Ind"() -> (w508:u16)
                  n157 = local read "Autorange Ind"() -> (w509:u16)
                  n158 = local read "Preferred Units Ind"() -> (w506:u16)
                  n159 = Format Into String(format string="INTYPE %s,%d,%d,%d,%d,%d,%d;", w512, w513, w510, w509, w508, 0, w506) -> (resulting string=w511:string)  [unwired: 2 in, 1 out]
                }
                event "Update Heater Settings": Value Change {
                  # "Generate settings command string"
                  n160 = event-data() -> ()  [unwired: 1 in, 2 out]
                  n161 = Format Into String(format string="SETP %s %d;", "1", "Heater Setpoint") -> (resulting string=w515:string)  [unwired: 2 in, 1 out]
                }
              }
              n162 = call "ReadLakeshoreSettings (SubVI).vi"("Prepended command"=w459, "error in (no error)"=w458, "Channel Str"=w444, "Lakeshore port"=w472) -> ("error out"=w449:errorcluster, "Settings array out"=w457:i32[], "VISA Refnum out"=w450:refnum<visa-resource-name>)  [unwired: 3 in]
              n163 = Index Array(array=w457) -> (element #1=w465:i32, element #2=w464:i32, element #3=w463:i32, element #4=w462:i32, element #5=w461:i32, element #6=w460:i32)  [unwired: 6 in]
              n164 = To Unsigned Word Integer(number=w465) -> (unsigned 16bit integer=w456:u16)
              "Excitation Mode Ind" <- w456
              n165 = To Unsigned Word Integer(number=w464) -> (unsigned 16bit integer=w455:u16)
              "Excitation Range Ind" <- w455
              n166 = To Unsigned Word Integer(number=w462) -> (unsigned 16bit integer=w453:u16)
              "Resistance Range Ind" <- w453
              n167 = To Unsigned Word Integer(number=w463) -> (unsigned 16bit integer=w454:u16)
              "Autorange Ind" <- w454
              n168 = To Unsigned Word Integer(number=w460) -> (unsigned 16bit integer=w451:u16)
              "Preferred Units Ind" <- w451
              n169 = Equal To 0?(x=w461) -> (x = 0?=w452:bool)
              "Excitation  Ind" <- w452
              n170 = case shown="True" w470 {
                tunnel: w451 -> [_ w524]
                tunnel: w452 -> [_ w523]
                tunnel: w453 -> [_ w522]
                tunnel: w454 -> [_ w521]
                tunnel: w455 -> [_ w520]
                tunnel: w456 -> [_ w519]
                frame False {
                }
                frame True {
                  n171 = local write "Autorange (0: Autorange off)"(w521) -> ()
                  n172 = local write "Preferred Units (2: Ohms)"(w524) -> ()
                  n173 = local write "Excitation Range"(w520) -> ()
                  n174 = local write "Resistance Range"(w522) -> ()
                  n175 = local write "Excitation  (T: On)"(w523) -> ()
                  n176 = local write "Excitation Mode"(w519) -> ()
                }
              }
              n177 = call "ReadHeaterSettings.vi"("error in (no error)"=w449, "VISA Refnum in"=w450) -> ("error out"=w448:errorcluster, "read buffer"=w446:string, "VISA Refnum out"=w447:refnum<visa-resource-name>)  [unwired: 7 in]
              n178 = local write "Heater Setpoint Ind"(w446) -> ()
            }
            frame #3 {
              # "Switchboard settings"
              # "Wait 50ms for safe comms to Lakeshore"
              n179 = event shown="[2] \"Open All IV\": Value Change" {
                selector: _ -> [_ _ _ _ _]
                dyn-events: _ -> [_ _ _ _ _]
                timeout: 50 -> [_ _ _ _ _]
                tunnel: [w538 w539 w551 w556 w567] -> w533
                tunnel: [w537 w542 w548 w555 w566] -> w532
                tunnel: w531 -> [w538 w544 w553 w560 w582]
                tunnel: w530 -> [w537 w543 w552 w559 w581]
                event Timeout {
                  n180 = event-data() -> ()  [unwired: 1 in, 3 out]
                }
                event "Open": Value Change {
                  # "Open channels on switchboard"
                  n181 = event-data() -> ()  [unwired: 1 in, 6 out]
                  n182 = local read "Channel Open/Close Array"() -> (w545:string)
                  n183 = Format Into String(format string="channel.open(\"%s\")", w545) -> (resulting string=w546:string)  [unwired: 2 in, 1 out]
                  n184 = VISA Write(VISA resource name=w544, write buffer=w546, error in (no error)=w543) -> (VISA resource name out=w541:refnum<visa-resource-name>, error out=w540:errorcluster)  [unwired: 1 out]
                  n185 = call <instrlib>:"ke37xx Error Query (Multiple).vi"("VISA resource name"=w541, "error in (no error)"=w540) -> ("VISA resource name out"=w539:refnum<visa-resource-name>, "error out"=w542:errorcluster)  [unwired: 10 in, 2 out]
                }
                event "Open All IV": Value Change {
                  # "Open all I-V channels on switchboard"
                  n186 = event-data() -> ()  [unwired: 1 in, 6 out]
                  n187 = VISA Write(VISA resource name=w553, write buffer="channel.open(\"1101:1414; 2101:2414\")", error in (no error)=w552) -> (VISA resource name out=w550:refnum<visa-resource-name>, error out=w549:errorcluster)  [unwired: 1 out]
                  n188 = call <instrlib>:"ke37xx Error Query (Multiple).vi"("VISA resource name"=w550, "error in (no error)"=w549) -> ("VISA resource name out"=w551:refnum<visa-resource-name>, "error out"=w548:errorcluster)  [unwired: 10 in, 2 out]
                }
                event "Close": Value Change {
                  # "Close specified channels on switchboard"
                  n189 = event-data() -> ()  [unwired: 1 in, 6 out]
                  n190 = local read "Channel Open/Close Array"() -> (w561:string)
                  n191 = Pick Line(multi-line string="channel.close(\"%s\")\nchannel.exclusiveclose(\"%s\")\nchannel.exclusiveslotclose(\"%s\")", line index=enum16{"Normal", "Exclusive", "Slot Exclusive"}."Normal" ("Mode (0: Normal)")) -> (output string=w562:string)  [unwired: 1 out]
                  n192 = Format Into String(format string=w562, w561) -> (resulting string=w564:string)  [unwired: 2 in, 1 out]
                  n193 = VISA Write(VISA resource name=w560, write buffer=w564, error in (no error)=w559) -> (VISA resource name out=w558:refnum<visa-resource-name>, error out=w557:errorcluster)  [unwired: 1 out]
                  n194 = call <instrlib>:"ke37xx Error Query (Multiple).vi"("VISA resource name"=w558, "error in (no error)"=w557) -> ("VISA resource name out"=w556:refnum<visa-resource-name>, "error out"=w555:errorcluster)  [unwired: 10 in, 2 out]
                }
                event "Lift pins (safe)": Value Change {
                  w573 = "channel.close(\"%s\")"
                  # "Open I-V pins"
                  # "Close common rail, then common-ground link"
                  n195 = event-data() -> ()  [unwired: 1 in, 1 out]
                  n196 = Format Into String(format string=w573, "1501:1512;2501:2512") -> (resulting string=w583:string)  [unwired: 2 in, 1 out]
                  n197 = VISA Write(VISA resource name=w582, write buffer=w583, error in (no error)=w581) -> (VISA resource name out=w578:refnum<visa-resource-name>, error out=w577:errorcluster)  [unwired: 1 out]
                  n198 = Format Into String(format string=w573, "1516,1616") -> (resulting string=w579:string)  [unwired: 2 in, 1 out]
                  n199 = VISA Write(VISA resource name=w578, write buffer=w579, error in (no error)=w577) -> (VISA resource name out=w576:refnum<visa-resource-name>, error out=w575:errorcluster)  [unwired: 1 out]
                  n200 = Format Into String(format string="channel.open(\"%s\")", "1101:1416; 2101:2416") -> (resulting string=w572:string)  [unwired: 2 in, 1 out]
                  n201 = VISA Write(VISA resource name=w576, write buffer=w572, error in (no error)=w575) -> (VISA resource name out=w569:refnum<visa-resource-name>, error out=w568:errorcluster)  [unwired: 1 out]
                  n202 = call <instrlib>:"ke37xx Error Query (Multiple).vi"("VISA resource name"=w569, "error in (no error)"=w568) -> ("VISA resource name out"=w567:refnum<visa-resource-name>, "error out"=w566:errorcluster)  [unwired: 10 in, 2 out]
                }
              }
              n203 = Wait (ms)(milliseconds to wait=50) -> ()  [unwired: 1 out]
            }
          }
          n204 = local read "Measurement\nperiod"() -> (w379:i64)
          n205 = Subtract(x=w349, y=0.5) -> (x-y=w348:dbl)
          n206 = node-c288(w379) -> ()  [unwired: 7 in, 1 out]
        }
      }
    }
    n207 = node-c288() -> ()  [unwired: 1 in, 1 out]
    n208 = node-c288() -> ()  [unwired: 1 in, 1 out]
  }
  "Array" <- w20
  "Graph indices out" <- w19
  n209 = node-c288(w60) -> ()  [unwired: 7 out]
  n210 = Bundle("VISA Refnum out"=w8, "error out"=w7, "Channel Str"=w6, "Channel Str"=w5, "VISA Refnum out"=w4, "VISA resource name out"=w3, "error out"=w2) -> (→"Comms out cluster":T9)  [unwired: 1 in]
